vi "New Report.vi"(8 "error in":errorcluster, 11 "connection reference":T1) -> (0 "error out":errorcluster, 3 "connection reference 2":T1)   [LabVIEW 2021]
uses:
  <vilib>/addons/database/Connection.llb/Conn ObjectReference.ctl
  <vilib>/addons/database/NI_Database_API.lvlib
panel:
  in  "stop":bool
  in  "Guardar":bool
  in  "AREA":string
  in  "MAQ":string
  in  "SOLUCION":string
  in  "DESCRIPCION":string
  # "CREAR NUEVO REPORTE"
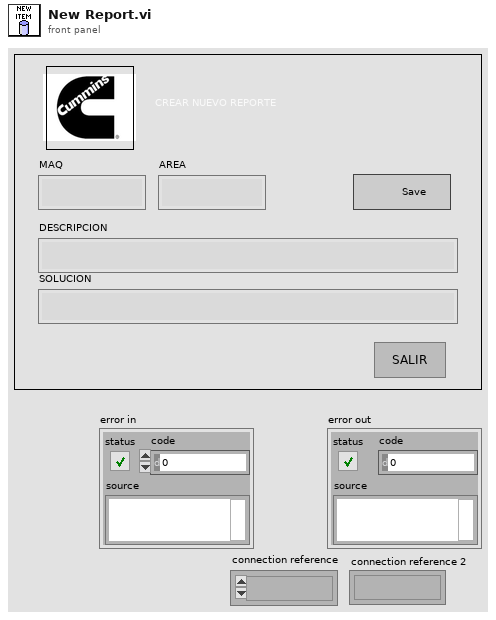
[diagram p1: front panel]
types:
  T1 = typedef "NI_Database_API.lvlib/Conn ObjectReference.ctl" = refnum<k1>
  T2 = enum8{"Enabled", "Disabled", "Disabled and Grayed Out"}
  T3 = cluster{"MAQ":string, "AREA":string, "DESCRIPCION":string, "SOLUCION":string, "date/time string":string}
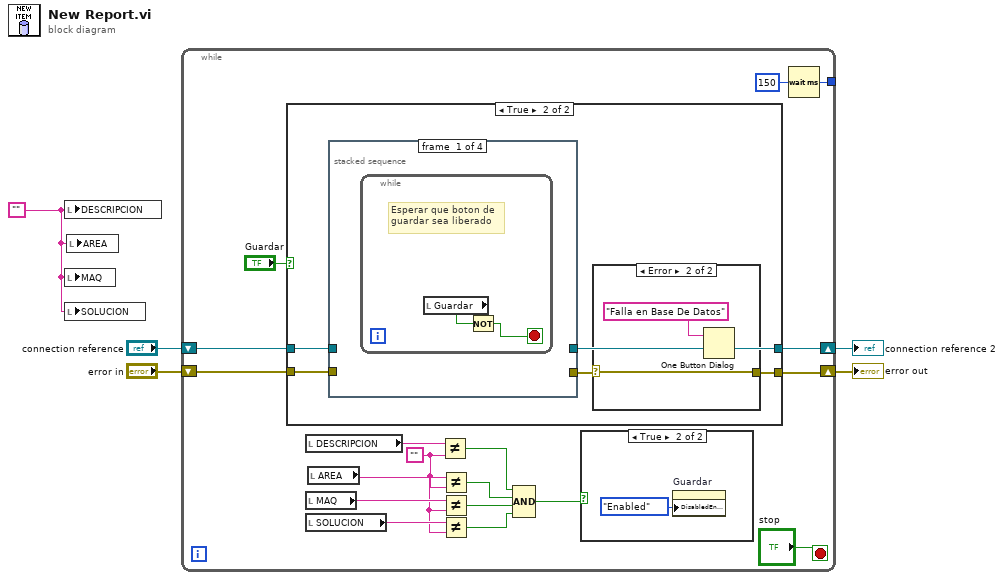
[diagram p0: block diagram]
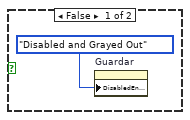
[diagram p2: hidden frame]
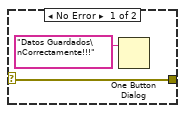
[diagram p4: hidden frame]
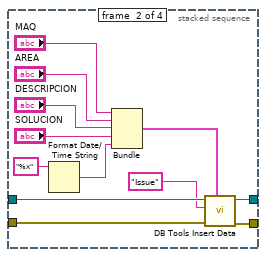
[diagram p5: hidden frame]
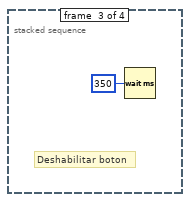
[diagram p6: hidden frame]
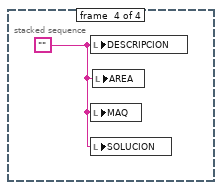
[diagram p7: hidden frame]
diagram:
  w1 = ""
  n1 = local write "DESCRIPCION"(w1) -> ()
  n2 = local write "MAQ"(w1) -> ()
  n3 = local write "SOLUCION"(w1) -> ()
  n4 = local write "AREA"(w1) -> ()
  n5 = while {
    shift-right: [w22] -> w2
    shift-left: "connection reference" -> [w23]
    shift-right: [w20] -> w3
    shift-left: "error in" -> [w21]
    tunnel: [w18] -> _
    stop <- "stop" stop-if-true
    w12 = ""
    n6 = case shown="True" "Guardar" {
      tunnel: w23 -> [w27 w32]
      tunnel: [w27 w31] -> w22
      tunnel: w21 -> [w26 w30]
      tunnel: [w26 w28] -> w20
      frame False {
      }
      frame True {
        n7 = stacked-sequence {
          tunnel: w32 -> [_ w50 _ _]
          tunnel: [_ w49 _ _] -> w31
          tunnel: w30 -> [_ w48 _ _]
          tunnel: [_ w47 _ _] -> w29
          frame #0 {
            n8 = while {
              stop <- w37 stop-if-true
              # "Esperar que boton de\nguardar sea liberado"
              n9 = local read "Guardar"() -> (w38:bool)
              n10 = Not(x=w38) -> (.not. x?=w37:bool)
            }
          }
          frame #1 {
            n11 = Format Date/Time String(time format string (%c)="%x") -> (date/time string=w39:string)  [unwired: 2 in]
            n12 = Bundle("MAQ"="MAQ", "AREA"="AREA", "DESCRIPCION"="DESCRIPCION", "SOLUCION"="SOLUCION", "date/time string"=w39) -> (w41:T3)  [unwired: 1 in]
            n13 = call <vilib>:"DB Tools Insert Data.vi"("data"=w41, "error in (no error)"=w48, "table"="Issue", "connection reference"=w50) -> ("error out"=w47:errorcluster, "connection reference out"=w49:T1)  [unwired: 6 in]
          }
          frame #2 {
            # "Deshabilitar boton"
            n14 = Wait (ms)(milliseconds to wait=u32 350) -> ()  [unwired: 1 out]
          }
          frame #3 {
            w52 = ""
            n15 = local write "DESCRIPCION"(w52) -> ()
            n16 = local write "MAQ"(w52) -> ()
            n17 = local write "SOLUCION"(w52) -> ()
            n18 = local write "AREA"(w52) -> ()
          }
        }
        n19 = case shown="Error" w29 {
          selector: w29 -> [w34 w36]
          tunnel: [w34 w36] -> w28
          frame No Error {
            n20 = One Button Dialog(message="Datos Guardados\nCorrectamente!!!") -> ()  [unwired: 1 in, 1 out]
          }
          frame Error {
            n21 = One Button Dialog(message="Falla en Base De Datos") -> ()  [unwired: 1 in, 1 out]
          }
        }
      }
    }
    n22 = local read "DESCRIPCION"() -> (w16:string)
    n23 = local read "MAQ"() -> (w14:string)
    n24 = local read "SOLUCION"() -> (w13:string)
    n25 = local read "AREA"() -> (w15:string)
    n26 = Not Equal?(x=w16, y=w12) -> (x != y?=w11:bool)
    n27 = Not Equal?(x=w15, y=w12) -> (x != y?=w10:bool)
    n28 = Not Equal?(x=w14, y=w12) -> (x != y?=w9:bool)
    n29 = Not Equal?(x=w13, y=w12) -> (x != y?=w8:bool)
    n30 = Compound Arithmetic op=AND(w11, w10, w9, w8) -> (w7:bool)
    n31 = case shown="True" w7 {
      frame False {
        n32 = property on="Guardar" class="Bool (strict)"("DisabledEnum"=T2."Disabled and Grayed Out" ("Disabled")) -> ()  [unwired: 2 in, 2 out]
      }
      frame True {
        n33 = property on="Guardar" class="Bool (strict)"("DisabledEnum"=T2."Enabled" ("Disabled")) -> ()  [unwired: 2 in, 2 out]
      }
    }
    n34 = Wait (ms)(milliseconds to wait=u32 150) -> (millisecond timer value=w18:u32)
  }
  "error out" <- w3
  "connection reference 2" <- w2
